vi "di.vi"(0 "RunMin":dbl, 1 "adjust":dbl=0.1, 2 "AD":dbl, 4 "Nvpai":dbl) -> (6 "Compensate1":dbl)   [LabVIEW 2018]
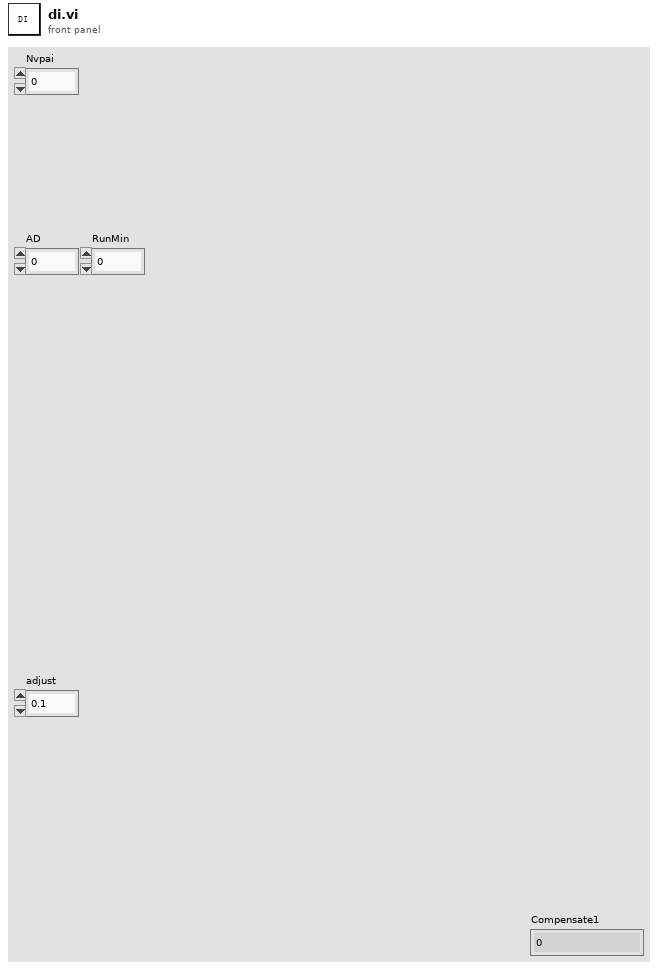
[diagram p1: front panel]
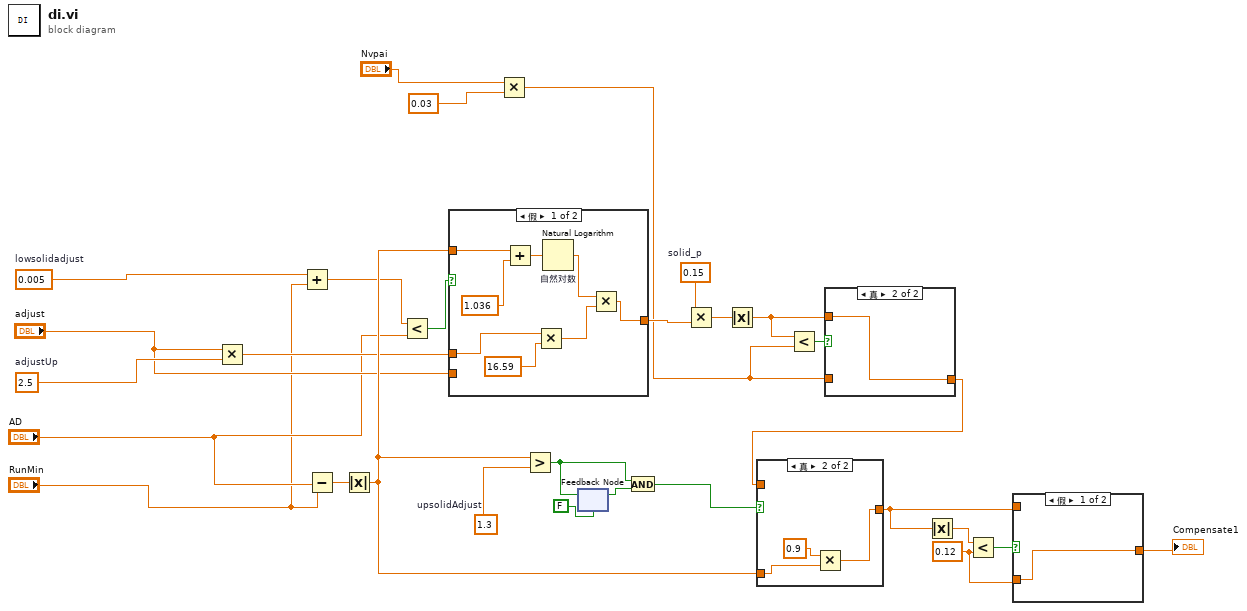
[diagram p0: block diagram]
diagram:
  w17 = 0.15  # solid_p
  w18 = 1.3  # upsolidAdjust
  w14 = 2.5  # adjustUp
  w12 = 0.005  # lowsolidadjust
  w9 = 0.12 ("RestrictAll")
  n1 = Multiply(x="adjust", y=w14) -> (x*y=w15:dbl)
  n2 = Add(x=w12, y="RunMin") -> (x+y=w11:dbl)
  n3 = Subtract(x="AD", y="RunMin") -> (x-y=w19:dbl)
  n4 = Absolute Value(x=w19) -> (abs(x)=w16:dbl)
  n5 = Less?(x=w11, y="AD") -> (x < y?=w22:bool)
  n6 = case shown="假" w22 {
    tunnel: [w37 w38] -> w21
    tunnel: w16 -> [w31 _]
    tunnel: "adjust" -> [_ w38]
    tunnel: w15 -> [w30 _]
    frame False {
      n7 = Add(x=w31, y=1.036) -> (x+y=w35:dbl)
      n8 = Multiply(x=w30, y=16.59) -> (x*y=w33:dbl)
      n9 = Natural Logarithm "自然对数"(1:w35) -> (0:w36:dbl)
      n10 = Multiply(x=w36, y=w33) -> (x*y=w37:dbl)
    }
    frame True {
    }
  }
  n11 = Multiply(x="Nvpai", y=0.03) -> (x*y=w4:dbl)
  n12 = Greater?(x=w16, y=w18) -> (0:w24:bool)
  n13 = feedback-in #1(w24) -> ()
  n14 = feedback #1(FALSE) -> (w25:bool)
  n15 = And(x=w24, y=w25) -> (x .and. y?=w26:bool)
  n16 = Multiply(x=w17, y=w21) -> (x*y=w28:dbl)
  n17 = Absolute Value(x=w28) -> (abs(x)=w20:dbl)
  n18 = Less?(x=w20, y=w4) -> (x < y?=w29:bool)
  n19 = case shown="真" w29 {
    tunnel: w20 -> [_ w40]
    tunnel: w4 -> [w39 _]
    tunnel: [w39 w40] -> w27
    frame False {
    }
    frame True {
    }
  }
  n20 = case shown="真" w26 {
    tunnel: [w41 w44] -> w7
    tunnel: w27 -> [w41 _]
    tunnel: w16 -> [_ w42]
    frame False {
    }
    frame True {
      n21 = Multiply(x=0.9 ("y"), y=w42) -> (x*y=w44:dbl)
    }
  }
  n22 = Absolute Value(x=w7) -> (abs(x)=w8:dbl)
  n23 = Less?(x=w8, y=w9) -> (x < y?=w10:bool)
  n24 = case shown="假" w10 {
    tunnel: w7 -> [_ w46]
    tunnel: w9 -> [w45 _]
    tunnel: [w45 w46] -> w6
    frame False {
    }
    frame True {
    }
  }
  "Compensate1" <- w6
